vi "Serial Sensor Read.vi"(6 "CO2 offset":dbl, 8 "error in (no error)":errorcluster, 11 "VISA resource name":refnum<visa-resource-name>) -> (0 "error out":errorcluster, 1 "Readings":T1, 2 "appended array":waveform(dbl)[](array[waveform]), 3 "VISA resource name out":refnum<visa-resource-name>)   [LabVIEW 2019]
doc: "This example performs a serial port write and a serial port read. The parameters set for the serial port must match the parameters of the connected instrument or device. The VISA Configure Serial Port VI sets the configuration parameters. The front panel displays the controls used to configure the basic parameters, such as baud rate, data bits, and parity. The VI passes the VISA resource name to other VIs that perform operations on that VISA resource. The VISA Write function sends a command to the serial device and the VISA Read function returns data based on the command. The VISA Close function then closes the reference to the serial device. It is important to close the reference; otherwise, further communication through that port might not be possible."
panel:
  out "Data Output":dbl[](array[numeric])
  # "Serial Sensor Read"
  # "(ppm)"
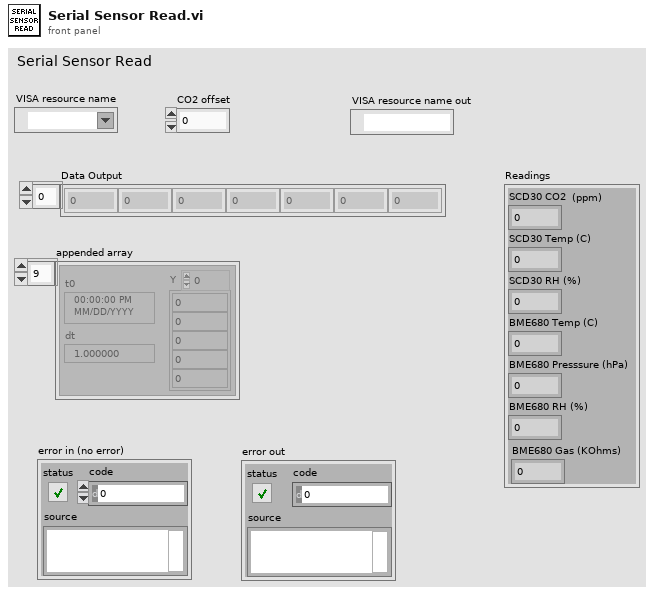
[diagram p1: front panel]
types:
  T1 = cluster{"SCD30 CO2":dbl, "SCD30 Temp (C)":dbl, "SCD30 RH (%)":dbl, "BME680 Temp (C) ":dbl, "BME680 Presssure (hPa)":dbl, "BME680 RH (%) ":dbl, "BME680 Gas (KOhms)":dbl}
  T2 = cluster{"Value":dbl, "Value":dbl, "Value":dbl, "Value":dbl, "Value":dbl, "Value":dbl, "Value":dbl}
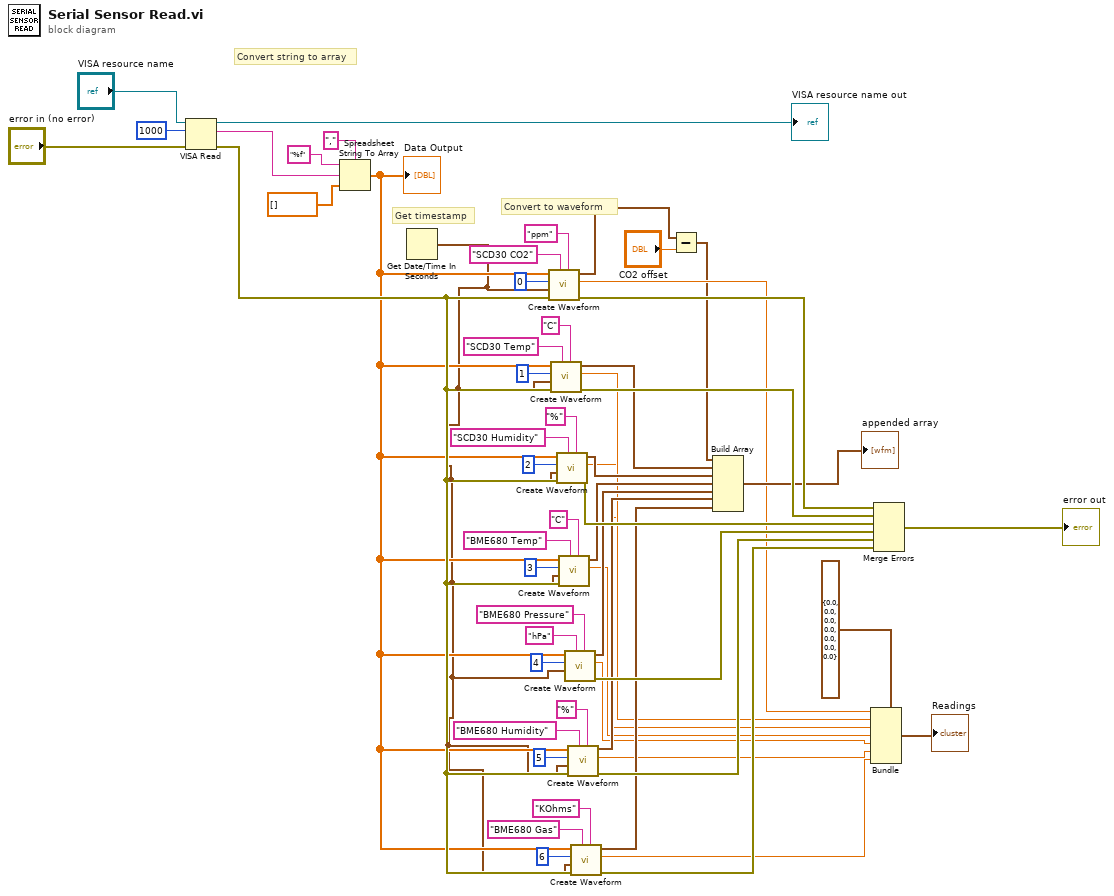
[diagram p0: block diagram]
diagram:
  # "Convert string to array"
  # "Convert to waveform"
  # "Get timestamp"
  n1 = VISA Read(VISA resource name="VISA resource name", byte count=u32 1000, error in (no error)="error in (no error)") -> (VISA resource name out=→"VISA resource name out":refnum<visa-resource-name>, read buffer=w56:string, error out=w31:errorcluster)  [unwired: 1 out]
  n2 = Spreadsheet String To Array(delimiter (Tab)=",", format string="%f", spreadsheet string=w56, array type (2D Dbl)=dbl[] []) -> (array=w17:dbl[])
  "Data Output" <- w17
  n3 = Get Date/Time In Seconds() -> (seconds since 1Jan1904=w4:timestamp)
  n4 = call "Create Waveform.vi"("Unit"="ppm", "Channel name"="SCD30 CO2", "error in (no error)"=w31, "t0"=w4, "index"=0, "array"=w17) -> ("error out"=w30:errorcluster, "Value"=w16:dbl, "output waveform"=w3:waveform(dbl))  [unwired: 3 in]
  n5 = call "Create Waveform.vi"("Unit"="C", "Channel name"="SCD30 Temp", "error in (no error)"=w31, "t0"=w4, "index"=1, "array"=w17) -> ("error out"=w29:errorcluster, "Value"=w15:dbl, "output waveform"=w24:waveform(dbl))  [unwired: 3 in]
  n6 = call "Create Waveform.vi"("Unit"="%", "Channel name"="SCD30 Humidity", "error in (no error)"=w31, "t0"=w4, "index"=2, "array"=w17) -> ("error out"=w28:errorcluster, "Value"=w14:dbl, "output waveform"=w23:waveform(dbl))  [unwired: 3 in]
  n7 = call "Create Waveform.vi"("Unit"="C", "Channel name"="BME680 Temp", "error in (no error)"=w31, "t0"=w4, "index"=3, "array"=w17) -> ("Value"=w13:dbl, "output waveform"=w22:waveform(dbl))  [unwired: 3 in, 1 out]
  n8 = call "Create Waveform.vi"("Unit"="BME680 Pressure", "Channel name"="hPa", "t0"=w4, "index"=4, "array"=w17) -> ("error out"=w27:errorcluster, "Value"=w12:dbl, "output waveform"=w21:waveform(dbl))  [unwired: 4 in]
  n9 = call "Create Waveform.vi"("Unit"="%", "Channel name"="BME680 Humidity", "error in (no error)"=w31, "t0"=w4, "index"=5, "array"=w17) -> ("error out"=w26:errorcluster, "Value"=w11:dbl, "output waveform"=w20:waveform(dbl))  [unwired: 3 in]
  n10 = call "Create Waveform.vi"("Unit"="KOhms", "Channel name"="BME680 Gas", "error in (no error)"=w31, "t0"=w4, "index"=6, "array"=w17) -> ("error out"=w25:errorcluster, "Value"=w10:dbl, "output waveform"=w19:waveform(dbl))  [unwired: 3 in]
  n11 = Subtract(x=w3, y="CO2 offset") -> (x-y=w2:waveform(dbl))
  n12 = Build Array(w2, w24, w23, w22, w21, w20, w19) -> (→"appended array":waveform(dbl)[])
  n13 = Bundle(cluster=T2 {"Value"=0.0, "Value"=0.0, "Value"=0.0, "Value"=0.0, "Value"=0.0, "Value"=0.0, "Value"=0.0}, "Value"=w16, "Value"=w15, "Value"=w14, "Value"=w13, "Value"=w12, "Value"=w11, "Value"=w10) -> (→"Readings":T2)
  n14 = Merge Errors(w30, w29, w28, w27, w26, w25) -> (→"error out":errorcluster)
